vi "Get Euler Angles.vi"(10 "Received Array":u8[](array[numeric]) format="%02x") -> (1 "Yaw (deg)":dbl, 2 "Pitch (deg)":dbl, 3 "Roll (deg)":dbl)   [LabVIEW 2012]
panel:
  # "7565800E0E0C3DFEFAD33E5CA4DA4031CF5E4033"
  # "7565 80 0E 0E 0C      3C3F7167    3D38044E     C0404563      446A\n7565800E0E0C3C3F655F3D381B48C04045E2C095\n7565800E0E0C3C3EB4673D37C64AC04045F1D1FC\n7565800E0E0C3C3EEC5A3D37C14AC04046070EB1\n7565800E0E0C3C3F2ACB3D378B53C040450F9810"
  # "75 65 80 0E 0E 0C 3C 3F 71 67 3D 38 04 4E C0 40 45 63 44 6A"
  # "YAW C0404563"
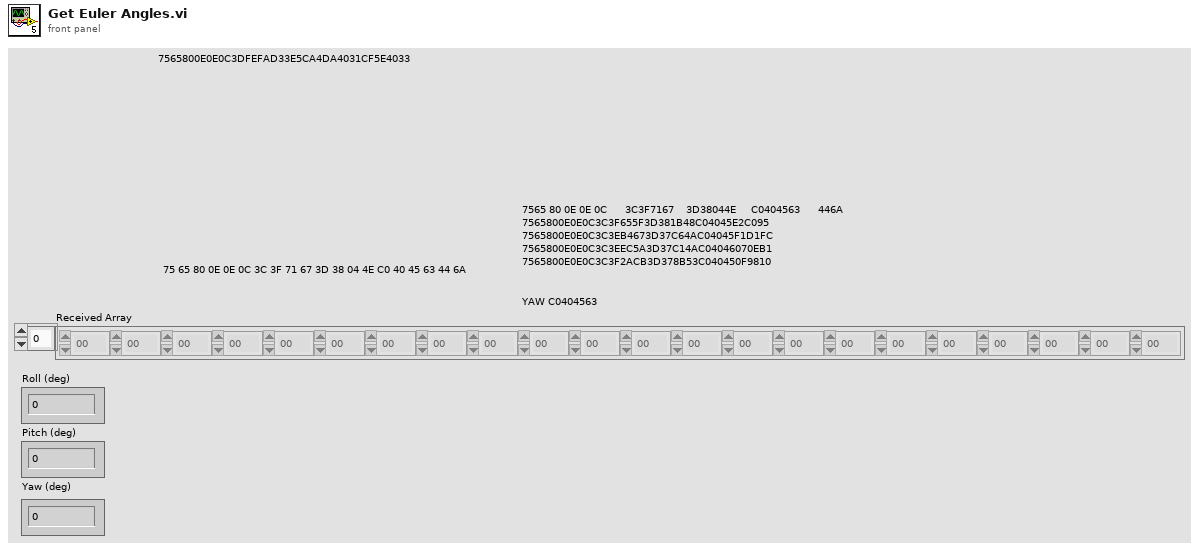
[diagram p1: front panel]
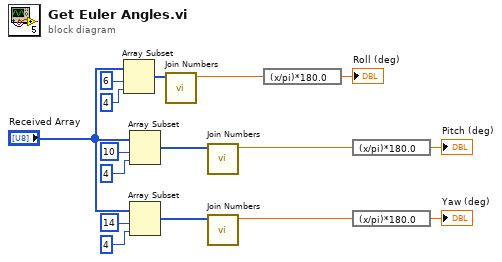
[diagram p0: block diagram]
diagram:
  n1 = Array Subset(array="Received Array", index=6, length=4) -> (w8:u8[])
  n2 = Array Subset(array="Received Array", index=10, length=4) -> (w10:u8[])
  n3 = Array Subset(array="Received Array", index=14, length=4) -> (w9:u8[])
  n4 = call "Join Numbers.vi"("Array of 4 U8"=w8) -> ("Single-Precision Float"=w6:sgl)  [unwired: 10 in]
  n5 = call "Join Numbers.vi"("Array of 4 U8"=w10) -> ("Single-Precision Float"=w1:sgl)  [unwired: 10 in]
  n6 = call "Join Numbers.vi"("Array of 4 U8"=w9) -> ("Single-Precision Float"=w4:sgl)  [unwired: 10 in]
  n7 = expression code="(x/pi)*180.0" ("radians to degrees")(w6) -> (→"Roll (deg)":sgl)
  n8 = expression code="(x/pi)*180.0" ("radians to degrees")(w1) -> (→"Pitch (deg)":sgl)
  n9 = expression code="(x/pi)*180.0" ("radians to degrees")(w4) -> (→"Yaw (deg)":sgl)
